vi "GRPCServerExample.vi"() -> ()   [LabVIEW 2019, in "MicronGRPCServer.lvlib"]
uses:
  Service/MicronGRPCServer.lvlib
  Service/GRPCService.lvclass
  <vilib>/Utility/error.llb/DialogType.ctl
  <vilib>/SLL Toolkit/SLL Queued State Machine/Queue Driver/Create Queue.vi
  <vilib>/SLL Toolkit/SLL Queued State Machine/Queue Driver/Enqueue an Item to Queue.vi
  <vilib>/SLL Toolkit/SLL Queued State Machine/Queue Driver/Dequeue Queue.vi
  <vilib>/SLL Toolkit/SLL Queued State Machine/Queue Driver/Enqueue N Items.vi
  <vilib>/SLL Toolkit/SLL Queued State Machine/Queue Driver/Flush Queue.vi
  <vilib>/SLL Toolkit/SLL Queued State Machine/Queue Driver/Release Queue.vi
  Base/Server/Message/MessageBase.lvclass
  <vilib>/SLL Toolkit/SLL Queued State Machine/SLL QSM.lvlib
  <vilib>/SLL Toolkit/SLL String/SLL String.lvlib
panel:
  out "Last Message Timestamp":string
  out "Payload":string
  out "Command":string
  in  "Connection String":string="localhost:50051"
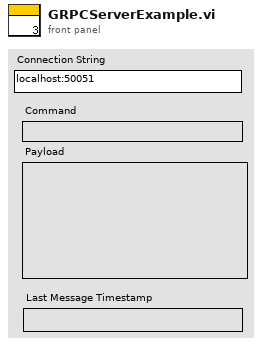
[diagram p1: front panel]
types:
  T1 = cluster{"Flags":cluster{"Source Code?":bool}, "GRPCServer":refnum<class "GRPCService.lvclass">}
  T2 = typedef "DialogType.ctl" = u16
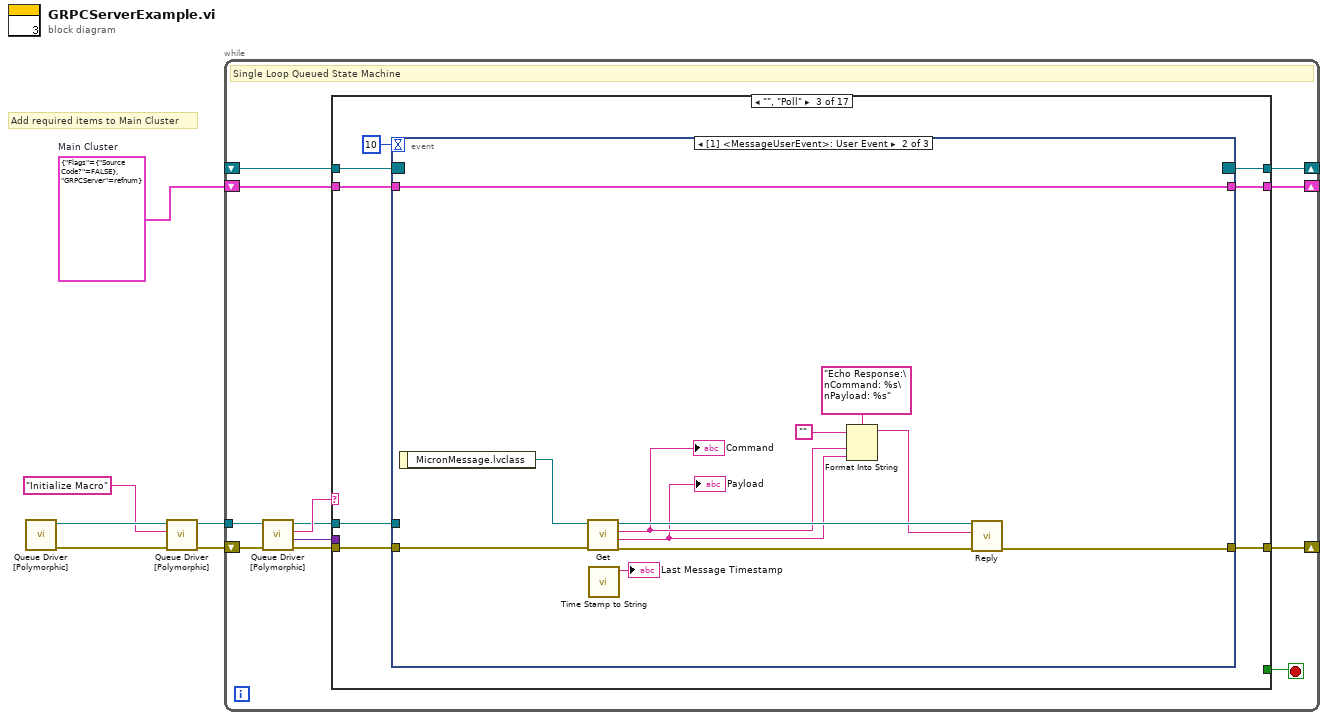
[diagram p0: block diagram]
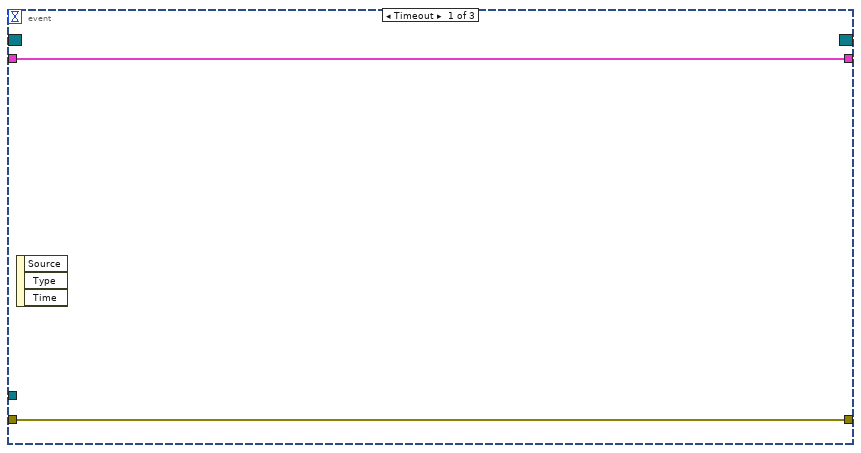
[diagram p4: hidden frame]
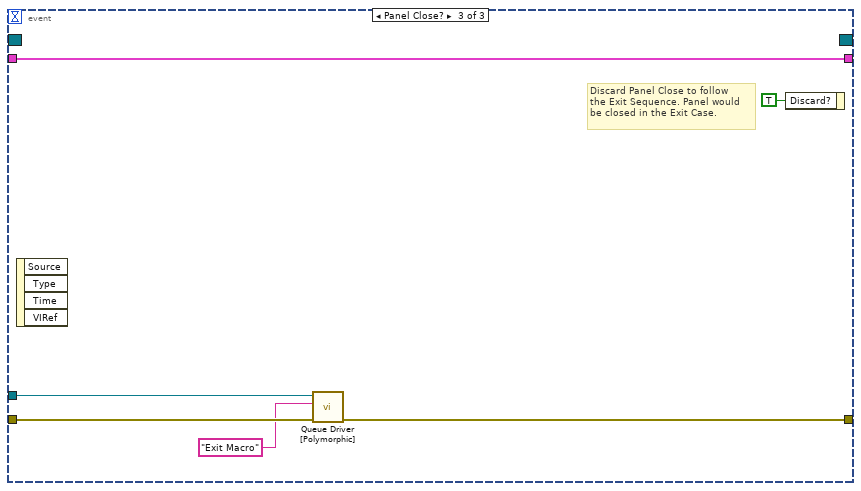
[diagram p5: hidden frame]
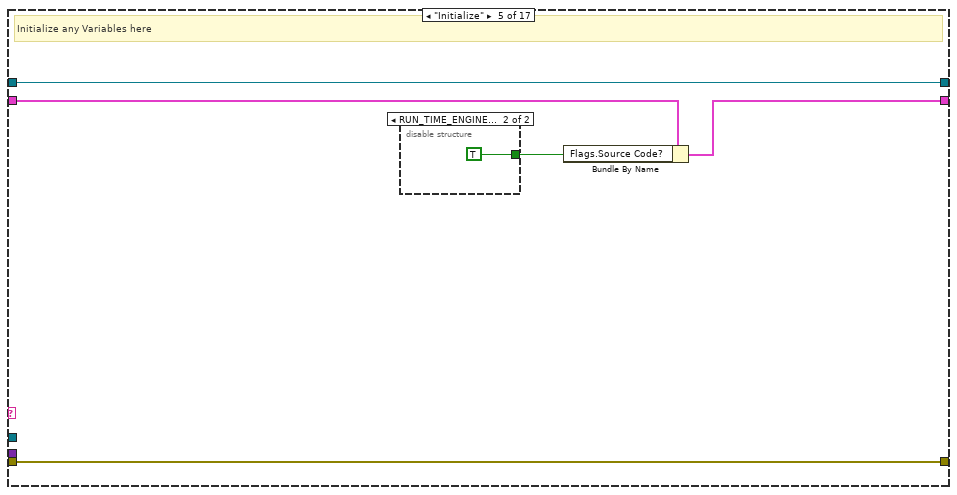
[diagram p7: hidden frame]
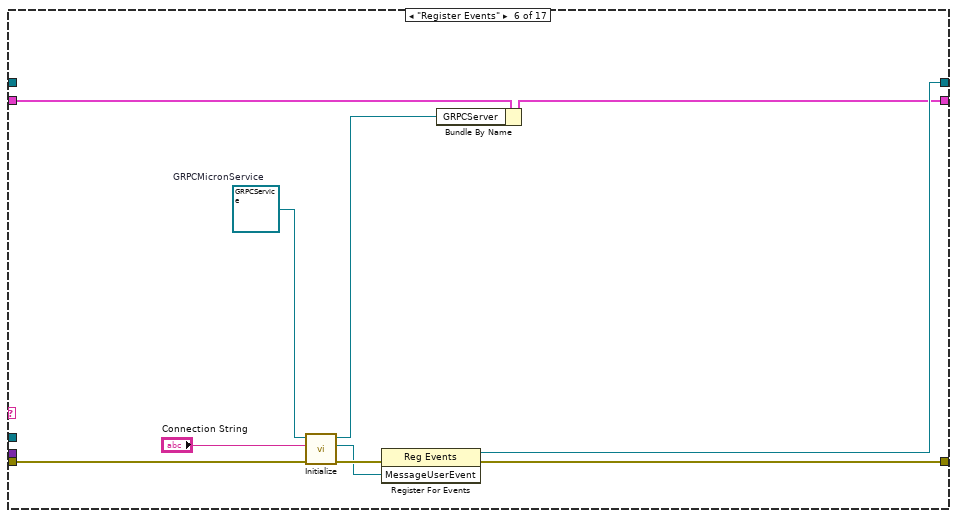
[diagram p9: hidden frame]
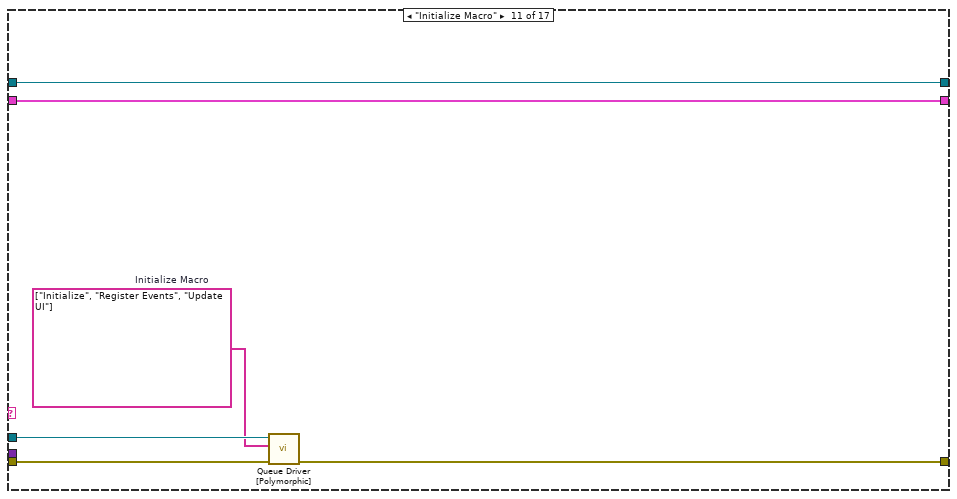
[diagram p14: hidden frame]
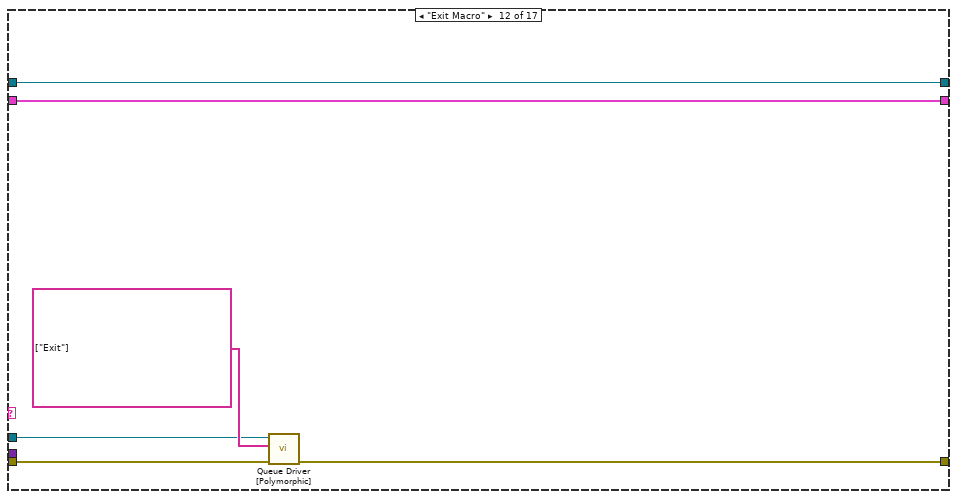
[diagram p15: hidden frame]
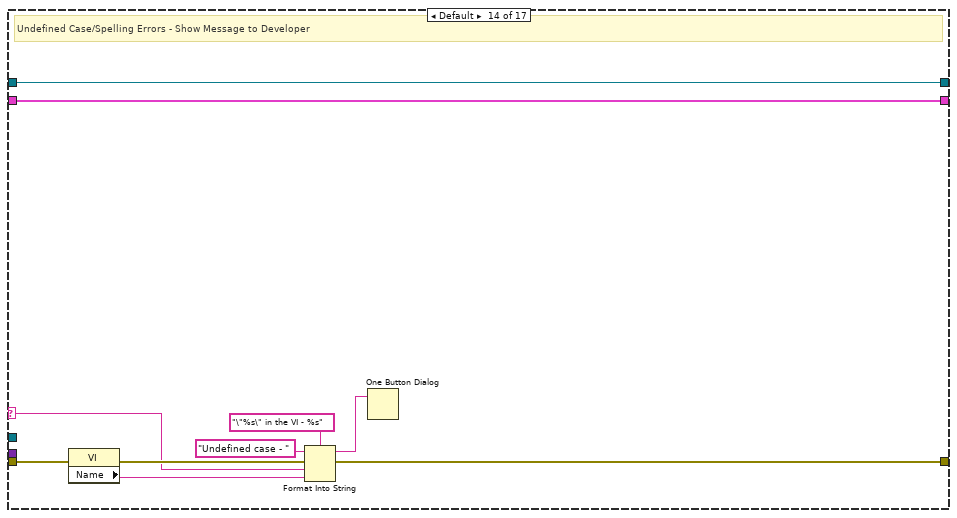
[diagram p17: hidden frame]
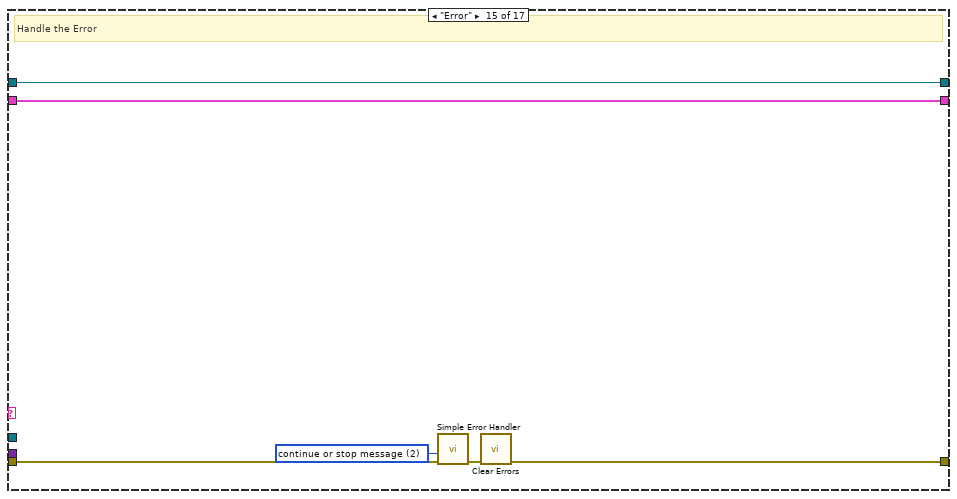
[diagram p18: hidden frame]
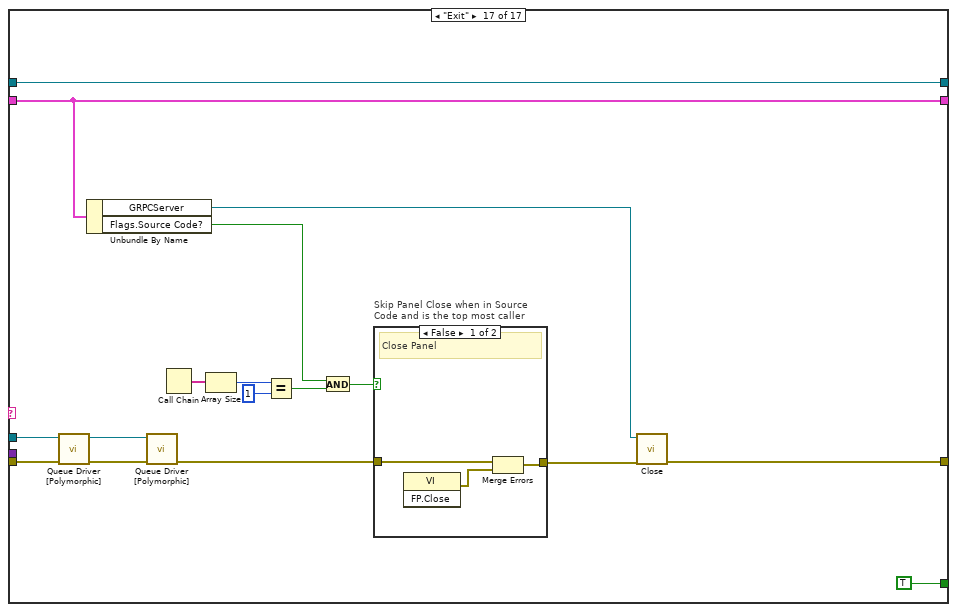
[diagram p20: hidden frame]
diagram:
  w3 = T1 {"Flags"={"Source Code?"=FALSE}, "GRPCServer"=refnum}  # Main Cluster
  # "Add required items to Main Cluster"
  n1 = call-poly <vilib>:"Queue Driver [Polymorphic].vi"() -> ("Error Out"=w1:errorcluster, "Queue Ref"=w5:refnum<queue>)  [unwired: 10 in]
  n2 = call-poly <vilib>:"Queue Driver [Polymorphic].vi"("Error In"=w1, "Item to Add"="Initialize Macro", "Queue Ref In"=w5) -> ("Error Out"=w2:errorcluster, "Queue Ref Out"=w6:refnum<queue>)  [unwired: 7 in]
  n3 = while "SLL Queued State Machine" {
    shift-right: [w16] -> _
    shift-left: w2 -> [w18]
    shift-right: [w14] -> _
    shift-left: _ -> [w13]
    shift-right: [w12] -> _
    shift-left: w3 -> [w11]
    tunnel: w6 -> [w9]
    stop <- w15 stop-if-true
    # "Single Loop Queued State Machine"
    n4 = call-poly <vilib>:"Queue Driver [Polymorphic].vi"("Error In"=w18, "Queue Ref In"=w9) -> ("Error Out"=w17:errorcluster, "Data"=w7:variant, "Dequeue"=w10:string, "Queue Ref Out"=w8:refnum<queue>)  [unwired: 6 in]
    n5 = case "QSM Case Structure" shown="\"\", \"Poll\"" w10 {
      selector: w10 -> [_ _ _ _ _ _ _ _ _ _ _ _ _ w99 _ _ _]
      tunnel: w17 -> [w21 w24 w30 w55 w60 w67 w74 w77 w80 w83 w87 w93 w98 w102 w114 w117 w132]
      tunnel: [w21 w24 w31 w55 w60 w71 w74 w77 w80 w83 w86 w92 w98 w105 w112 w117 w120] -> w16
      tunnel: [_ _ _ _ _ _ _ _ _ _ _ _ _ _ _ _ TRUE] -> w15
      tunnel: [w20 w23 w29 w54 w59 w70 w73 w76 w79 w82 w89 w95 w97 w108 w111 w116 w131] -> w14
      tunnel: w13 -> [w20 w23 w28 w54 w59 _ w73 w76 w79 w82 w89 w95 w97 w108 w111 w116 w131]
      tunnel: [w19 w22 w26 w53 w56 w64 w72 w75 w78 w81 w88 w94 w96 w107 w110 w115 w130] -> w12
      tunnel: w11 -> [w19 w22 w27 w53 w57 w69 w72 w75 w78 w81 w88 w94 w96 w107 w110 w115 w130]
      tunnel: w8 -> [_ _ w25 _ _ _ _ _ _ _ w85 w90 _ _ _ _ w122]
      tunnel: w7 -> [_ _ _ _ _ _ _ _ _ _ _ _ _ _ _ _ _]
      frame "/--------------- Read Me -----------------/" {
        # "General Purpose Queue Based State Machine for Any Use Case (main application, module, pop up message etc)\n\nAdvantages:\n1. Lean Project Code Base (dependencies are in vilib).\n2. This template can be safely used in multiple parallel running modules without any issues.\n3. This template can also be safely used even in cases where the VI is configured to be a clone, where multiple \ninstances of the VI could be executing concurrently.\n\nHow to Use:\n1. Add necessary items to the Main Cluster.\n2. Use the Polymorphic Queue Driver for doing any queue operations. \n3. Add any required user events in the \"Register Events\" case. Ignore if not needed.\n4. Use \"Macros\" section for defining any list of state calls, which could be used in multiple places. \nEx: Initialize Macro, might be needed if we need to any reinitialization."
      }
      frame "/------------------ Poll -------------------/" {
      }
      frame "", "Poll" {
        n6 = event shown="[1] <MessageUserEvent>: User Event" {
          selector: w28 -> [_ _ _]
          dyn-events: [_ _ _] -> w29
          timeout: 10 -> [_ _ _]
          tunnel: [w34 w41 w51] -> w31
          tunnel: w30 -> [w34 w44 w52]
          tunnel: w27 -> [w33 w46 w50]
          tunnel: [w33 w46 w50] -> w26
          tunnel: w25 -> [_ _ w48]
          event Timeout {
            n7 = event-data() -> ()  [unwired: 1 in, 3 out]
          }
          event User Event {
            n8 = event-data() -> ("MicronMessage.lvclass"=w45:refnum<class "MessageBase.lvclass">)  [unwired: 1 in]
            n9 = call-dynamic "Get.vi"("error in (no error)"=w44, "MicronMessage in"=w45) -> ("error out"=w43:errorcluster, "Payload"=w38:string, "Command"=w39:string, "MicronMessage out"=w42:refnum<class "MessageBase.lvclass">)  [unwired: 6 in]
            "Command" <- w39
            "Payload" <- w38
            n10 = call <vilib>:"Time Stamp to String.vi"() -> ("Output String"=→"Last Message Timestamp":string)  [unwired: 11 in]
            n11 = Format Into String(format string="Echo Response:\nCommand: %s\nPayload: %s", initial string="", w39, w38) -> (resulting string=w36:string)  [unwired: 1 in, 1 out]
            n12 = call-dynamic "Reply.vi"("error in (no error)"=w43, "Response"=w36, "MicronMessage in"=w42) -> ("error out"=w41:errorcluster)  [unwired: 7 in, 1 out]
          }
          event Panel Close? {
            # "Discard Panel Close to follow\nthe Exit Sequence. Panel would\nbe closed in the Exit Case."
            n13 = event-data() -> ()  [unwired: 1 in, 4 out]
            n14 = call-poly <vilib>:"Queue Driver [Polymorphic].vi"("Error In"=w52, "Item to Add"="Exit Macro" ("Enqueue"), "Queue Ref In"=w48) -> ("Error Out"=w51:errorcluster)  [unwired: 7 in, 1 out]
            n15 = event-data("Discard?"=TRUE) -> ()  [unwired: 1 in, 1 out]
          }
        }
      }
      frame "/--------------- Initialize -----------------/" {
      }
      frame "Initialize" {
        # "Initialize any Variables here"
        n16 = disable-structure shown="RUN_TIME_ENGINE==False" {
          disable-tunnel: [_ TRUE] -> w58
          frame condition #0 {
          }
          frame condition #1 (active) {
          }
        }
        n17 = Bundle By Name(cluster=w57, "Flags.Source Code?"=w58) -> (w56:T1)
      }
      frame "Register Events" {
        w65 = refnum<class "GRPCService.lvclass"> refnum  # GRPCMicronService
        n18 = call-dynamic "Initialize.vi"("error in (no error)"=w67, "Connection String"="Connection String", "MicronServer in"=w65) -> ("error out"=w68:errorcluster, "MessageUserEvent"=w66:refnum<user-event>, "MicronServer out"=w63:refnum<class "GRPCService.lvclass">)  [unwired: 6 in]
        n19 = register-events(error in=w68, w66) -> (reference out=w70:refnum<event-registration>, error out=w71:errorcluster)  [unwired: 1 in]
        n20 = Bundle By Name(cluster=w69, "GRPCServer"=w63) -> (w64:T1)
      }
      frame "/---------- Custom Case Splitter ----------/" {
      }
      frame "/-------------- User Interface --------------/" {
        # "Duplicate this case to create additional case splitters for readability"
      }
      frame "Update UI" {
        # "Update Front Panel Controls in this Case"
      }
      frame "/----------------- Macros -----------------/" {
      }
      frame "Initialize Macro" {
        w84 = string[] ["Initialize", "Register Events", "Update UI"]  # Initialize Macro
        n21 = call-poly <vilib>:"Queue Driver [Polymorphic].vi"("Error In"=w87, "Enqueue N"=w84, "Queue Ref In"=w85) -> ("Error Out"=w86:errorcluster)  [unwired: 7 in, 1 out]
      }
      frame "Exit Macro" {
        n22 = call-poly <vilib>:"Queue Driver [Polymorphic].vi"("Error In"=w93, "Enqueue N"=string[] ["Exit"], "Queue Ref In"=w90) -> ("Error Out"=w92:errorcluster)  [unwired: 7 in, 1 out]
      }
      frame "/-------------- Error Handler--------------/" {
      }
      frame Default {
        # "Undefined Case/Spelling Errors - Show Message to Developer"
        n23 = property class="VI"(error in=w102) -> (error out=w101:errorcluster, "Name"=w100:string)  [unwired: 1 in, 1 out]
        n24 = Format Into String(format string="\"%s\" in the VI - %s" ("message"), initial string="Undefined case - ", error in=w101, w99, w100) -> (resulting string=w103:string, error out=w105:errorcluster)
        n25 = One Button Dialog(message=w103) -> ()  [unwired: 1 in, 1 out]
      }
      frame "Error" {
        w109 = T2 2 items=["no dialog", "OK message", "continue or stop message", "OK message + warnings", "continue/stop + warnings"] ("type of dialog (OK msg:1)")
        # "Handle the Error"
        n26 = call <vilib>:"Simple Error Handler.vi"("type of dialog (OK msg:1)"=w109, "error in (no error)"=w114) -> ("error out"=w113:errorcluster)  [unwired: 3 in, 4 out]
        n27 = call <vilib>:"Clear Errors.vi"("error in (no error)"=w113) -> ("error out"=w112:errorcluster)  [unwired: 5 in, 1 out]
      }
      frame "/------------------- Exit --------------------/" {
      }
      frame "Exit" {
        n28 = call-poly <vilib>:"Queue Driver [Polymorphic].vi"("Error In"=w132, "Queue Ref In"=w122) -> ("Error Out"=w133:errorcluster, "Queue Ref Out"=w121:refnum<queue>)  [unwired: 7 in, 1 out]
        n29 = Unbundle By Name(w130) -> ("GRPCServer"=w118:refnum<class "GRPCService.lvclass">, "Flags.Source Code?"=w124:bool)
        n30 = call-poly <vilib>:"Queue Driver [Polymorphic].vi"("Error In"=w133, "Queue Ref In"=w121) -> ("Error Out"=w129:errorcluster)  [unwired: 9 in]
        n31 = Call Chain() -> (call chain=w128:string[])
        n32 = Array Size(array=w128) -> (size(s)=w127:i32)
        n33 = Equal?(x=w127, y=1) -> (x = y?=w125:bool)
        n34 = And(x=w124, y=w125) -> (x .and. y?=w123:bool)
        n35 = case "Skip Panel Close when in Source\nCode and is the top most caller" shown="False" w123 {
          tunnel: w129 -> [w136 w138]
          tunnel: [w137 w138] -> w119
          frame False {
            # "Close Panel"
            n36 = invoke class="VI" method="FP.Close"() -> (error out=w135:errorcluster)  [unwired: 3 in, 2 out]
            n37 = Merge Errors(w136, w135) -> (w137:errorcluster)
          }
          frame True {
            # "Do Not Close Panel"
          }
        }
        n38 = call-dynamic "Close.vi"("error in (no error)"=w119, "MicronServer in"=w118) -> ("error out"=w120:errorcluster)  [unwired: 8 in, 1 out]
      }
    }
  }
